vi "Actor Core.vi"(8 "error in":errorcluster, 11 "Nested in":refnum<class "Display_Console_UI.lvclass">) -> (0 "error out":errorcluster, 3 "Actor out":refnum<class "Actor.lvclass">)   [LabVIEW 2025, in "Display_Console_UI.lvlib" / "Display_Console_UI.lvclass"]
doc: "(<B>Filename</B>: Actor Framework.lvlib:Actor.lvclass:Actor Core.vi)\n\nReceives messages to the actor, reacts to them, and initiates any error handling that may shut the actor down.\n\nDescendant classes may override this VI to append parallel tasks for the actor to complete while it handles messages. Overrides use the Call Parent Method node."
uses:
  Display_Console_UI.lvclass
  Display_Console_UI.lvclass/Display_Console_UI.ctl
  <vilib>/ActorFramework/Actor/Actor.lvclass
  <vilib>/ActorFramework/Stop Msg/Stop Msg.lvclass
panel:
  out "DISPLAY":string
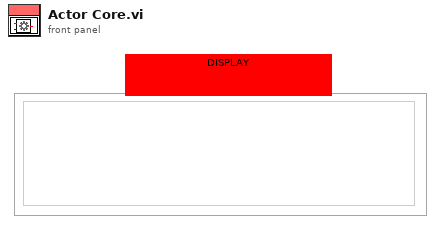
[diagram p1: front panel]
types:
  T1 = cluster{"Stop":refnum<user-event>, "Display":refnum<user-event>}
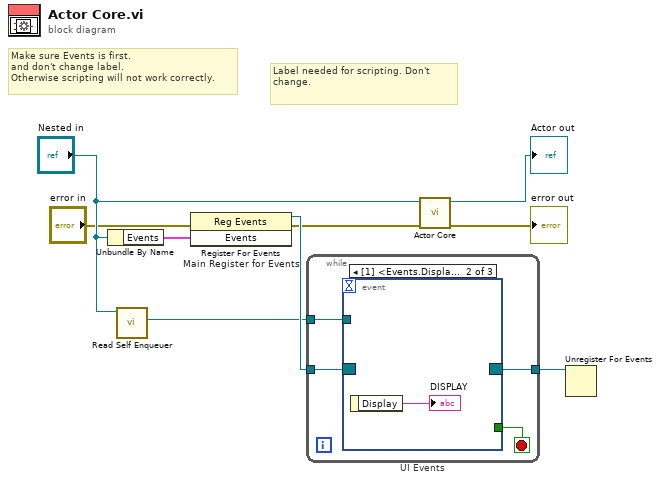
[diagram p0: block diagram]
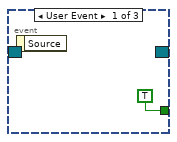
[diagram p2: hidden frame]
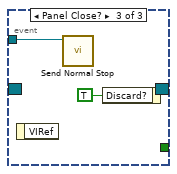
[diagram p3: hidden frame]
diagram:
  # "Label needed for scripting. Don't change."
  # "Make sure Events is first.\nand don't change label.\nOtherwise scripting will not work correctly."
  n1 = Unbundle By Name("Nested in") -> ("Events"=w1:T1)
  n2 = call <vilib>:"Read Self Enqueuer.vi"("Actor"="Nested in") -> ("Self Enqueuer"=w4:refnum<class "Message Enqueuer.lvclass">)  [unwired: 10 in]
  n3 = register-events "Main Register for Events"(error in="error in", w1) -> (reference out=w7:refnum<event-registration>, error out=w2:errorcluster)  [unwired: 1 in]
  n4 = while {
    tunnel: w7 -> [w13]
    tunnel: [w11] -> w6
    tunnel: w4 -> [w10]
    stop <- w12 stop-if-true
    n5 = event "UI Events" shown="[1] <Events.Display>: User Event" {
      selector: w13 -> [_ _ _]
      dyn-events: [_ _ _] -> w11
      timeout: _ -> [_ _ _]
      tunnel: [TRUE _ _] -> w12
      tunnel: w10 -> [_ _ w16]
      event User Event {
        n6 = event-data() -> ()  [unwired: 1 in, 1 out]
      }
      event User Event {
        n7 = event-data() -> ("Display"=→"DISPLAY":string)  [unwired: 1 in]
      }
      event Panel Close? {
        n8 = event-data() -> ()  [unwired: 1 in, 1 out]
        n9 = call <vilib>:"Send Normal Stop.vi"("Message Enqueuer"=w16) -> ()  [unwired: 10 in, 1 out]
        n10 = event-data("Discard?"=TRUE) -> ()  [unwired: 1 in, 1 out]
      }
    }
  }
  n11 = call-parent "Actor Core.vi"("error in"=w2, "Actor in"="Nested in") -> ("error out"=→"error out":errorcluster, "Actor out"=→"Actor out":refnum<class "Actor.lvclass">)  [unwired: 8 in]
  n12 = Unregister For Events(event registration refnum=w6) -> ()  [unwired: 1 in, 1 out]
